vi "Update Channel UI.vi"(8 "error in (no error)":errorcluster, 10 "Channels":T1[][](array[typedef]), 11 "CIF_UI in":refnum<class "CIF_Manager_UI.lvclass">) -> (0 "error out":errorcluster, 3 "CIF_UI out":refnum<class "CIF_Manager_UI.lvclass">)   [LabVIEW 2021, in "CIF_Manager_UI.lvclass"]
uses:
  CIF_Manager_UI.lvclass
  <vilib>/CIF Foundation/CIF Core/CIFCore/Grpc/CIFCoreChannel_client/RPC Messages/cif_management_common_Channel.ctl
  <vilib>/CIF Foundation/CIF Core/CIFCore/Grpc/CIFCoreChannel_client/RPC Messages/cif_management_common_ChannelDirection.ctl
  <vilib>/CIF Foundation/CIF Core/CIFCore/Grpc/CIFCoreChannel_client/RPC Messages/cif_management_common_ChannelPattern.ctl
  CIF_Manager_UI.lvclass/CIF_Manager_UI.ctl
  <vilib>/CIF Foundation/CIF Core/CIFUI/Typedef/Direction to Include.ctl
  <vilib>/CIF Foundation/CIF Core/CIFUI/CIF_UI.lvclass
  <vilib>/CIF Foundation/CIF Core/CIFCore/Grpc/CIFCoreChannel_client/CIFCoreChannel_client.lvlib
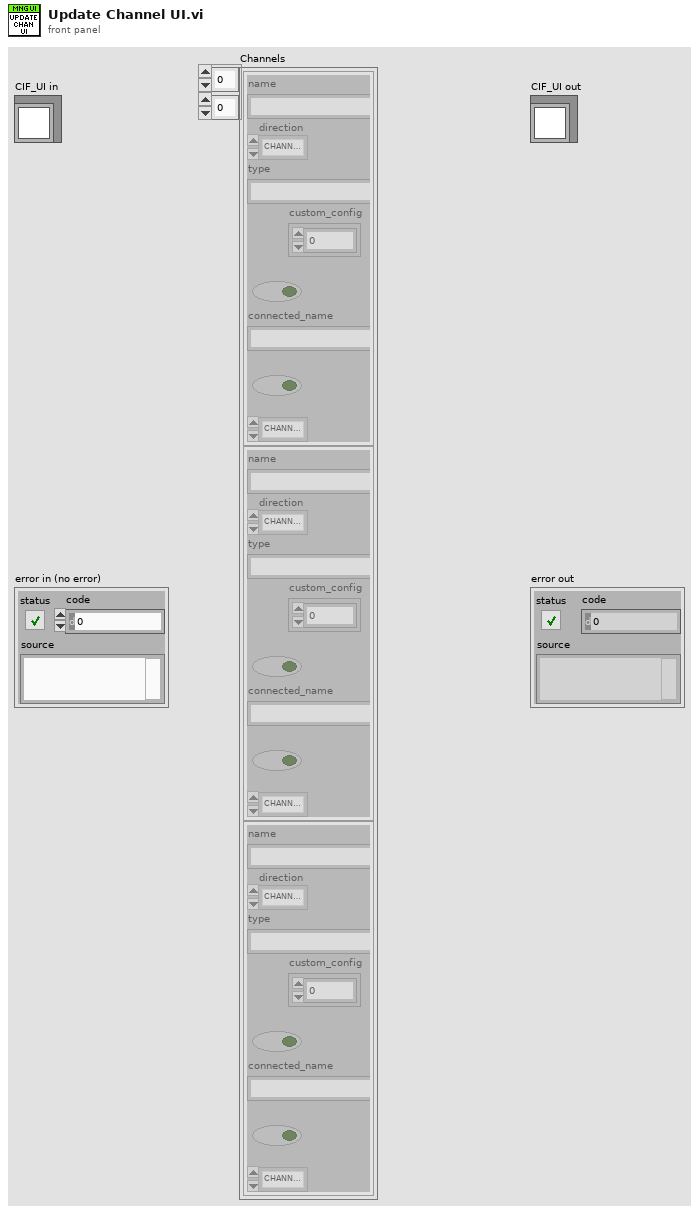
[diagram p1: front panel]
types:
  T1 = typedef "CIFCoreChannel_client.lvlib/cif_management_common_Channel.ctl" = cluster{"name":string, "direction":T2, "type":string, "custom_config":u8[], "connected":bool, "connected_name":string, "forced":bool, "channel_pattern":T3}
  T2 = typedef "CIFCoreChannel_client.lvlib/cif_management_common_ChannelDirection.ctl" = enum32{"CHANNELDIRECTION_UNKNOWN", "CHANNELDIRECTION_PUBLISHER", "CHANNELDIRECTION_SUBSCRIBER"}
  T3 = typedef "CIFCoreChannel_client.lvlib/cif_management_common_ChannelPattern.ctl" = enum32{"CHANNELPATTERN_UNKNOWN", "CHANNELPATTERN_TAG", "CHANNELPATTERN_FIFO", "CHANNELPATTERN_MULTIFIFO", "CHANNELPATTERN_BACKPRESSUREFIFO"}
  T4 = typedef "CIF_UI.lvclass/Direction to Include.ctl" = enum16{"All", "Subscriber", "Publisher"}
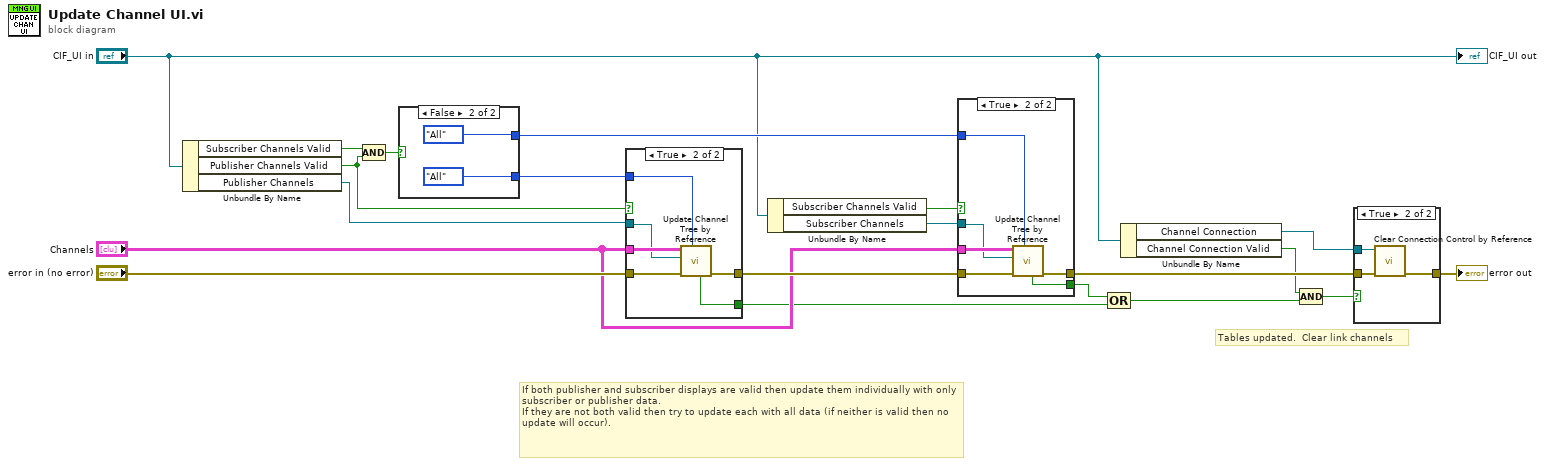
[diagram p0: block diagram]
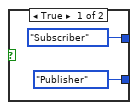
[diagram p3: hidden frame]
diagram:
  # "Tables updated.  Clear link channels"
  # "If both publisher and subscriber displays are valid then update them individually with only subscriber or publisher data.  \nIf they are not both valid then try to update each with all data (if neither is valid then no update will occur)."
  n1 = Unbundle By Name("CIF_UI in") -> ("Subscriber Channels Valid"=w20:bool, "Publisher Channels Valid"=w12:bool, "Publisher Channels"=w11:refnum<vi>)
  n2 = Compound Arithmetic op=AND(w20, w12) -> (w15:bool)
  n3 = case shown="False" w15 {
    tunnel: [Direction_to_Include."Subscriber" ("Direction to Include") Direction_to_Include."All" ("Direction to Include")] -> w13
    tunnel: [Direction_to_Include."Publisher" ("Direction to Include") Direction_to_Include."All" ("Direction to Include")] -> w14
    frame True {
    }
    frame False {
    }
  }
  n4 = case shown="True" w12 {
    tunnel: "Channels" -> [_ w31]
    tunnel: w11 -> [_ w30]
    tunnel: w14 -> [_ w29]
    tunnel: "error in (no error)" -> [w25 w28]
    tunnel: [w25 w27] -> w17
    tunnel: [_ w26] -> w9
    frame False {
    }
    frame True {
      n5 = call <vilib>:"Update Channel Tree by Reference.vi"("Direction to Include"=w29, "error in (no error)"=w28, "Channnel Tree ref in"=w30, "Channels"=w31) -> ("error out"=w27:errorcluster, "Update"=w26:bool)  [unwired: 6 in]
    }
  }
  n6 = Unbundle By Name("CIF_UI in") -> ("Subscriber Channels Valid"=w18:bool, "Subscriber Channels"=w19:refnum<vi>)
  n7 = case shown="True" w18 {
    tunnel: "Channels" -> [_ w38]
    tunnel: w19 -> [_ w37]
    tunnel: w13 -> [_ w36]
    tunnel: w17 -> [w32 w35]
    tunnel: [w32 w34] -> w7
    tunnel: [_ w33] -> w8
    frame False {
    }
    frame True {
      n8 = call <vilib>:"Update Channel Tree by Reference.vi"("Direction to Include"=w36, "error in (no error)"=w35, "Channnel Tree ref in"=w37, "Channels"=w38) -> ("error out"=w34:errorcluster, "Update"=w33:bool)  [unwired: 6 in]
    }
  }
  n9 = Compound Arithmetic op=OR(w8, w9) -> (w4:bool)
  n10 = Unbundle By Name("CIF_UI in") -> ("Channel Connection"=w2:refnum<vi>, "Channel Connection Valid"=w3:bool)
  n11 = Compound Arithmetic op=AND(w3, w4) -> (w1:bool)
  n12 = case shown="True" w1 {
    tunnel: w7 -> [w39 w42]
    tunnel: [w39 w41] -> w6
    tunnel: w2 -> [_ w40]
    frame False {
    }
    frame True {
      n13 = call "Clear Connection Control by Reference.vi"("error in"=w42, "Channel Connection"=w40) -> ("error out"=w41:errorcluster)  [unwired: 9 in]
    }
  }
  "error out" <- w6
  "CIF_UI out" <- "CIF_UI in"
